vi "Can_File_be_Editted.vi"(0 "Filename":path) -> (1 "File Permissions OK?":bool, 2 "File Status":T1=enum."Directory structure cannot be created", 3 "Comment String":string="Directory structure cannot be created", 4 "Cannot create directory":path)   [LabVIEW 2018]
uses:
  File_Status.ctl
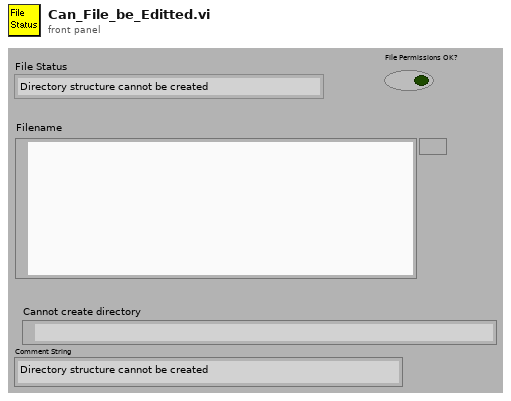
[diagram p1: front panel]
types:
  T1 = typedef "File_Status.ctl" = enum16{"Invalid Path", "File Does not Exist", "This is a folder pathname", "Generic File Error", "Directory structure cannot be created", "File cannot be created", "File can be created", "File exist but read only", "File exist but no access", "File exist with read and write access"}
  T2 = enum16{"read/write", "read-only", "write-only", "write-only (truncate)"}
  T3 = enum16{"open", "replace", "create", "open or create", "replace or create", "replace or create with confirmation"}
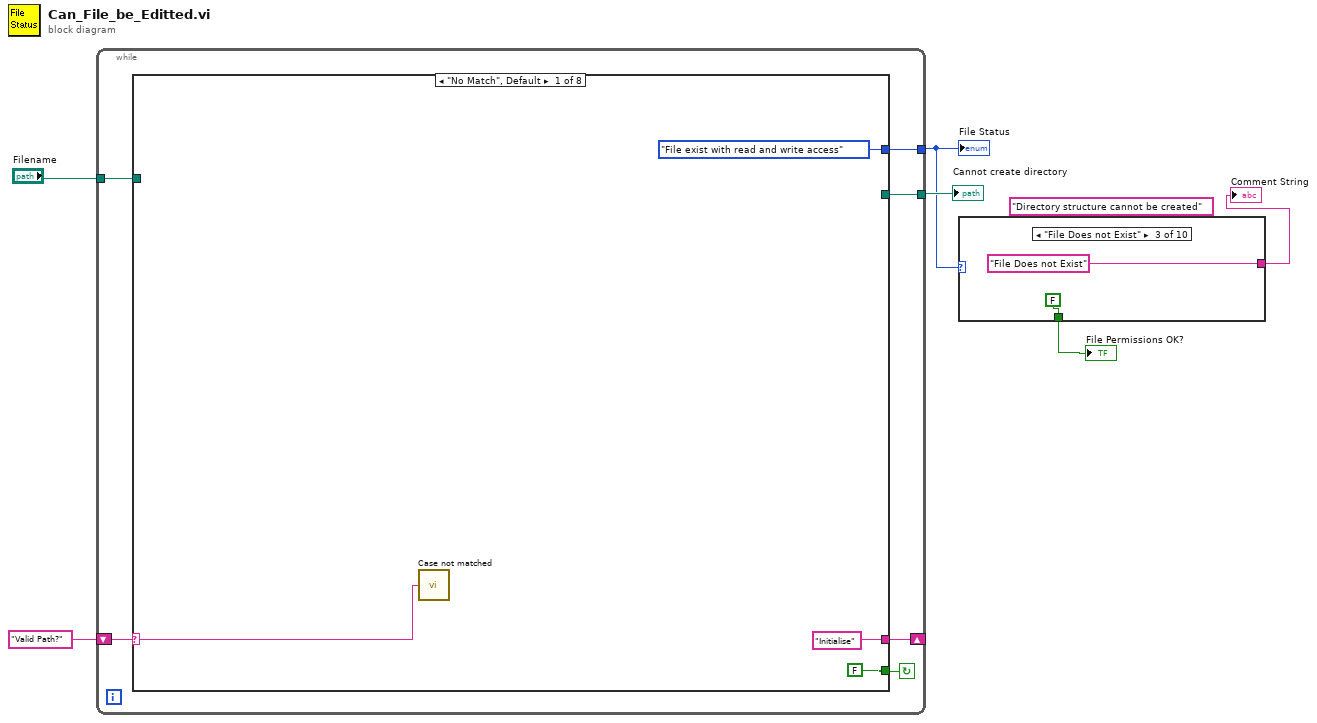
[diagram p0: block diagram]
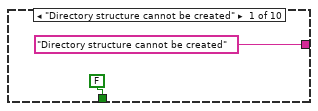
[diagram p2: hidden frame]
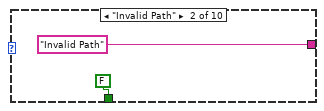
[diagram p3: hidden frame]
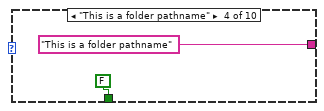
[diagram p4: hidden frame]
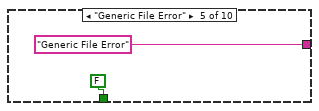
[diagram p5: hidden frame]
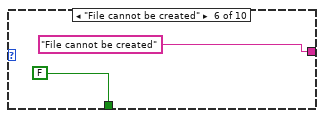
[diagram p6: hidden frame]
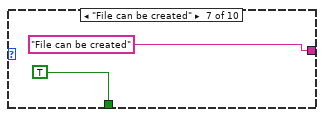
[diagram p7: hidden frame]
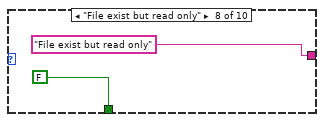
[diagram p8: hidden frame]
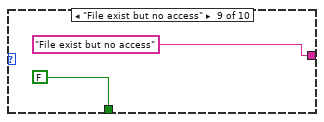
[diagram p9: hidden frame]
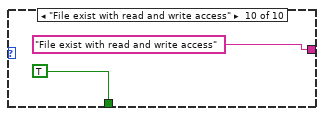
[diagram p10: hidden frame]
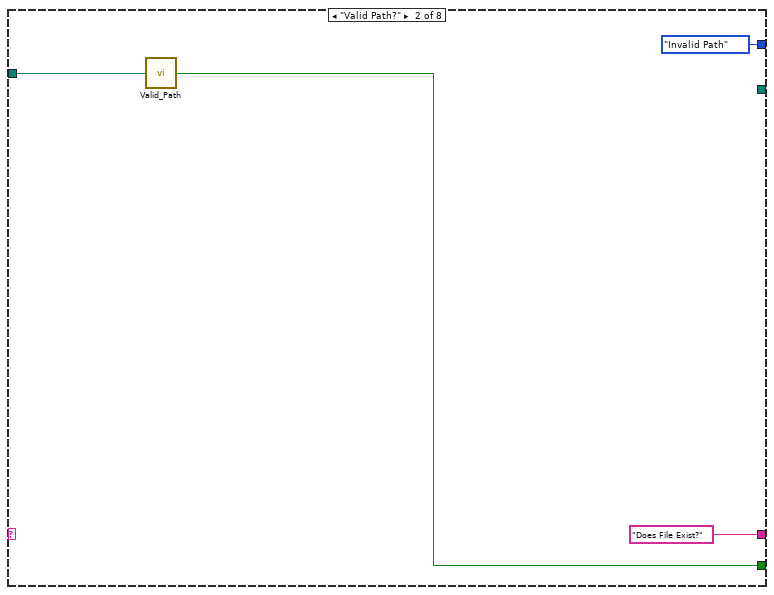
[diagram p11: hidden frame]
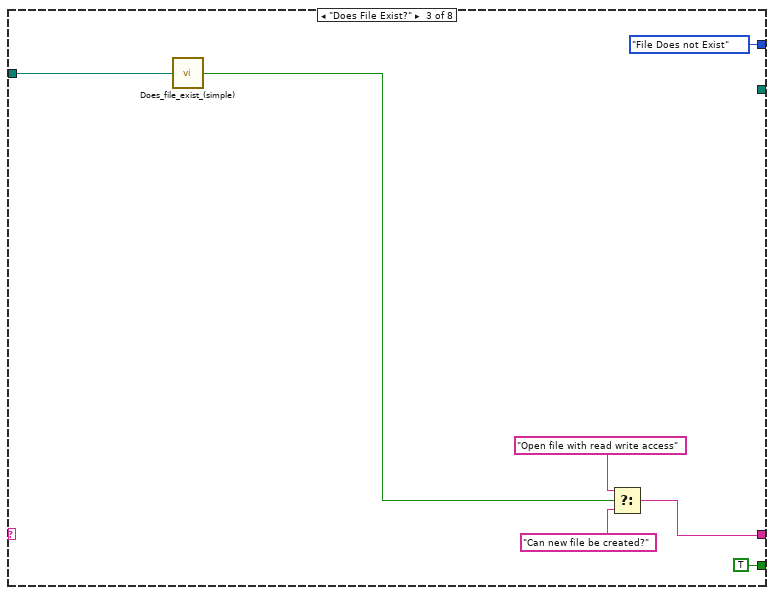
[diagram p12: hidden frame]
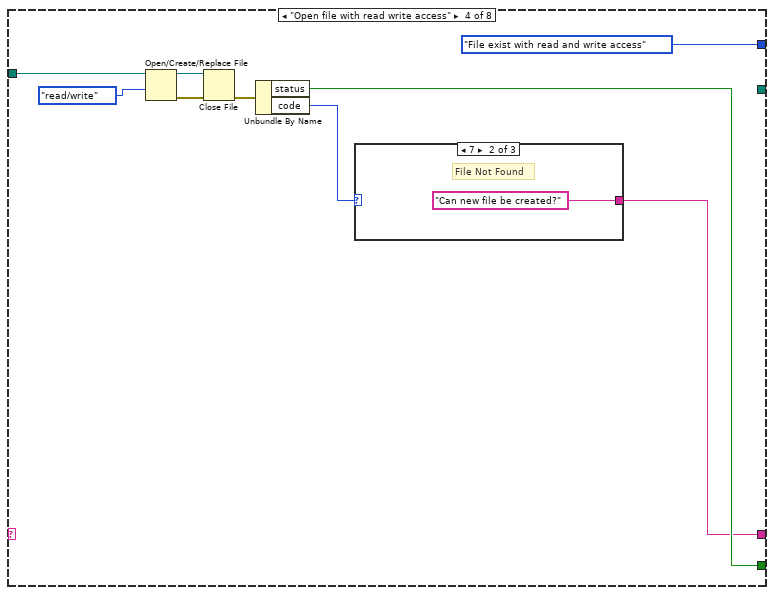
[diagram p13: hidden frame]
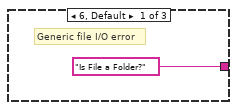
[diagram p14: hidden frame]
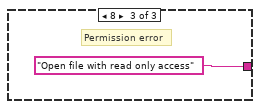
[diagram p15: hidden frame]
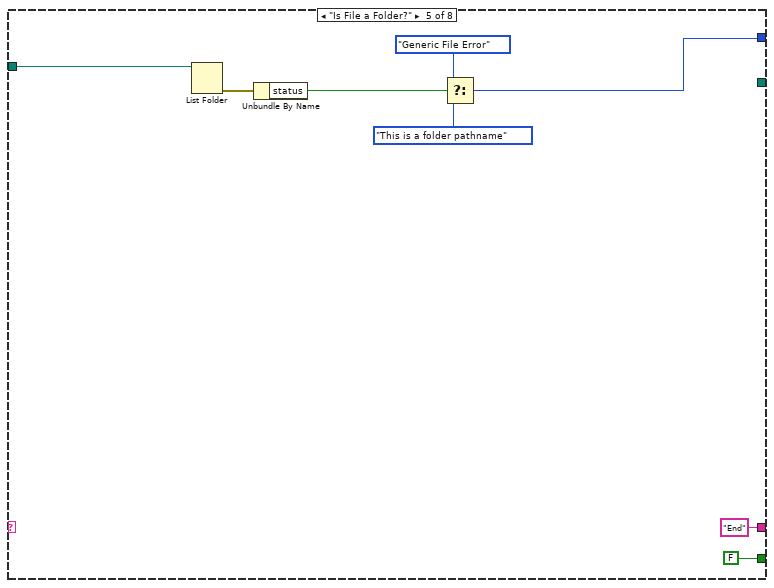
[diagram p16: hidden frame]
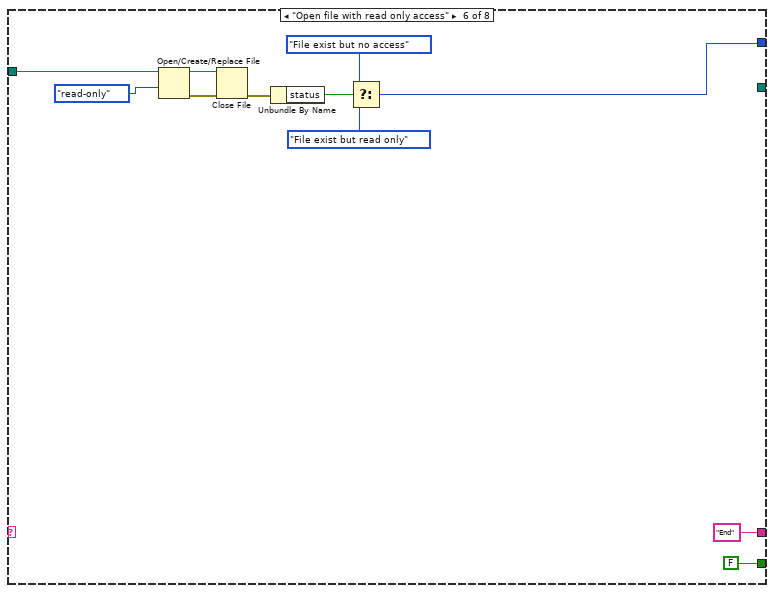
[diagram p17: hidden frame]
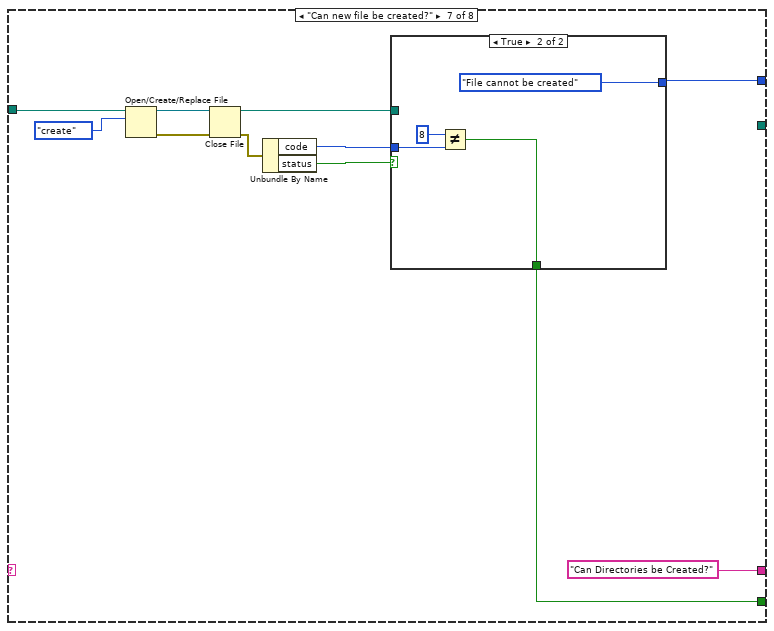
[diagram p18: hidden frame]
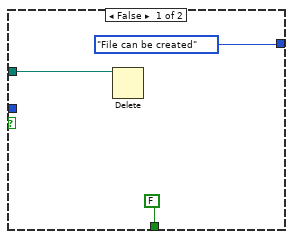
[diagram p19: hidden frame]
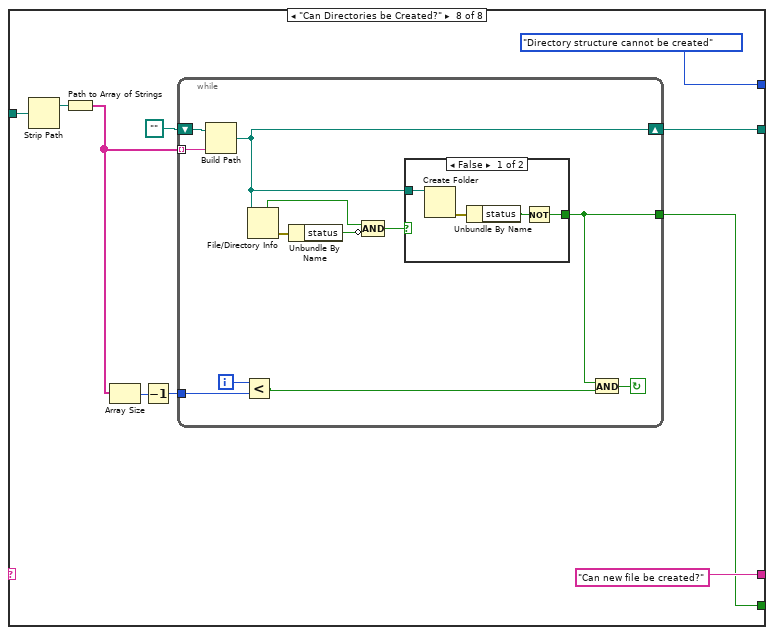
[diagram p20: hidden frame]
diagram:
  (unwired) "Directory structure cannot be created"
  n1 = while {
    shift-left: "Valid Path?" -> [w10]
    shift-right: [w11] -> _
    tunnel: "Filename" -> [w9]
    tunnel: [w8] -> w4
    tunnel: [w7] -> w5
    stop <- w12 continue-if-true
    n2 = case shown="\"No Match\", Default" w10 {
      selector: w10 -> [w13 _ _ _ _ _ _ _]
      tunnel: [FALSE w18 TRUE ("status") w31 FALSE ("status") FALSE ("status") w62 w78] -> w12
      tunnel: ["Initialise" "Does File Exist?" w22 w28 "End" ("f") "End" "Can Directories be Created?" "Can new file be created?"] -> w11
      tunnel: w9 -> [_ w19 w26 w33 w47 w53 w64 w84]
      tunnel: [File_Status."File exist with read and write access" ("File Status") File_Status."Invalid Path" ("File Status") File_Status."File Does not Exist" ("File Status") File_Status."File exist with read and write access" ("File Status") w40 w48 w60 File_Status."Directory structure cannot be created" ("File Status")] -> w8
      tunnel: [_ _ _ _ _ _ _ w77] -> w7
      frame "No Match", Default {
        n3 = call "Case not matched.vi"("Case Name not Matched"=w13) -> ()
      }
      frame "Valid Path?" {
        n4 = call "Valid_Path.vi"("Filename"=w19) -> ("Valid Path?"=w18:bool)
      }
      frame "Does File Exist?" {
        n5 = call "Does_file_exist_(simple).vi"("Pathname"=w26) -> ("exists?"=w24:bool)
        n6 = Select(t="Open file with read write access", s=w24, f="Can new file be created?") -> (s? t:f=w22:string)
      }
      frame "Open file with read write access" {
        n7 = Open/Create/Replace File(file path (use dialog)=w33, access (0:read/write)=T2."read/write" ("open mode (0)")) -> (refnum out=w34:refnum<file>, error out=w36:errorcluster)  [unwired: 1 in, 4 out]
        n8 = Close File(refnum=w34, error in=w36) -> (error out=w30:errorcluster)  [unwired: 1 out]
        n9 = Unbundle By Name(w30) -> ("status"=w31:bool, "code"=w29:i32)
        n10 = case shown="7" w29 {
          tunnel: ["Is File a Folder?" ("f") "Can new file be created?" ("f") "Open file with read only access"] -> w28
          frame 6, Default {
            # "Generic file I/O error"
          }
          frame 7 {
            # "File Not Found"
          }
          frame 8 {
            # "Permission error"
          }
        }
      }
      frame "Is File a Folder?" {
        n11 = List Folder(path=w47) -> (error out=w46:errorcluster)  [unwired: 1 in, 5 out]
        n12 = Unbundle By Name(w46) -> ("status"=w43:bool)
        n13 = Select(t=File_Status."Generic File Error" ("File Status"), s=w43, f=File_Status."This is a folder pathname" ("File Status")) -> (s? t:f=w40:T1)
      }
      frame "Open file with read only access" {
        n14 = Open/Create/Replace File(file path (use dialog)=w53, access (0:read/write)=T2."read-only" ("open mode (0)")) -> (refnum out=w54:refnum<file>, error out=w57:errorcluster)  [unwired: 1 in, 4 out]
        n15 = Close File(refnum=w54, error in=w57) -> (error out=w56:errorcluster)  [unwired: 1 out]
        n16 = Unbundle By Name(w56) -> ("status"=w51:bool)
        n17 = Select(t=File_Status."File exist but no access" ("File Status"), s=w51, f=File_Status."File exist but read only" ("File Status")) -> (s? t:f=w48:T1)
      }
      frame "Can new file be created?" {
        n18 = Open/Create/Replace File(file path (use dialog)=w64, operation (0:open)=T3."create") -> (refnum out=w68:refnum<file>, error out=w67:errorcluster)  [unwired: 1 in, 4 out]
        n19 = Close File(refnum=w68, error in=w67) -> (path=w63:path, error out=w66:errorcluster)
        n20 = Unbundle By Name(w66) -> ("code"=w61:i32, "status"=w65:bool)
        n21 = case shown="True" w65 {
          tunnel: w63 -> [w72 _]
          tunnel: [FALSE w73] -> w62
          tunnel: w61 -> [_ w76]
          tunnel: [File_Status."File can be created" ("File Status") File_Status."File cannot be created" ("File Status")] -> w60
          frame False {
            n22 = Delete(path (use dialog)=w72) -> ()  [unwired: 1 in, 6 out]
          }
          frame True {
            n23 = Not Equal?(x=8, y=w76) -> (x != y?=w73:bool)
          }
        }
      }
      frame "Can Directories be Created?" {
        n24 = Strip Path(path=w84) -> (stripped path=w79:path)  [unwired: 1 out]
        n25 = Path to Array of Strings(0:w79) -> (2:w81:string[])  [unwired: 1 out]
        n26 = Array Size(array=w81) -> (size(s)=w83:i32)
        n27 = Decrement(x=w83) -> (x-1=w82:i32)
        n28 = while {
          tunnel: [w93] -> w78
          tunnel: w82 -> [w96]
          shift-left: path "" ("appended path") -> [w98]
          shift-right: [w92] -> w77
          tunnel: w81 -> [w97] mode=indexing
          i -> [w87]
          stop <- w94 continue-if-true
          n29 = Build Path(base path=w98, name or relative path=w97) -> (appended path=w92:path)
          n30 = Less?(x=w87, y=w96) -> (x < y?=w95:bool)
          n31 = File/Directory Info(path=w92) -> (directory=w89:bool, error out=w91:errorcluster)  [unwired: 1 in, 5 out]
          n32 = Unbundle By Name(w91) -> ("status"=w90:bool)
          n33 = Compound Arithmetic op=AND(w89, invert w90) -> (w88:bool)
          n34 = case shown="False" w88 {
            tunnel: w92 -> [w102 _]
            tunnel: [w99 TRUE] -> w93
            frame False {
              n35 = Create Folder(path (use dialog)=w102) -> (error out=w101:errorcluster)  [unwired: 1 in, 3 out]
              n36 = Unbundle By Name(w101) -> ("status"=w100:bool)
              n37 = Not(x=w100) -> (.not. x?=w99:bool)
            }
            frame True {
            }
          }
          n38 = And(x=w93, y=w95) -> (x .and. y?=w94:bool)
        }
      }
    }
  }
  "File Status" <- w4
  "Cannot create directory" <- w5
  n39 = case shown="\"File Does not Exist\"" w4 {
    tunnel: [FALSE FALSE FALSE FALSE FALSE FALSE TRUE FALSE FALSE TRUE] -> w3
    tunnel: ["Directory structure cannot be created" "Invalid Path" "File Does not Exist" "This is a folder pathname" "Generic File Error" "File cannot be created" "File can be created" "File exist but read only" "File exist but no access" "File exist with read and write access"] -> w2
    frame "Directory structure cannot be created" {
    }
    frame "Invalid Path" {
    }
    frame "File Does not Exist" {
    }
    frame "This is a folder pathname" {
    }
    frame "Generic File Error" {
    }
    frame "File cannot be created" {
    }
    frame "File can be created" {
    }
    frame "File exist but read only" {
    }
    frame "File exist but no access" {
    }
    frame "File exist with read and write access" {
    }
  }
  "File Permissions OK?" <- w3
  "Comment String" <- w2
